vi "Execute Subscription Policy.vi"(9 "Publish Time":timestamp, 10 "New Topic Value":variant, 11 "Subscription Policy":T1) -> (0 "error out (Unsubscribe?)":errorcluster, 3 "Subscription Policy Out":T1)   [LabVIEW 2017, in "IMediator.lvlib" / "ISubscriptionPolicy.lvclass"]
doc: "This method decides whether or not to send or otherwise handle the new data value. The policy is set and maintained by the subscriber. The Topic Actor knows no policy details, it just passes the new value in. If there is a failure inside this method, the Topic Actor must assume the listener is no longer valid (dead/unrecoverable) and should delete it from the Subscriber list.\n\n<License>\nCopyright © 2017 Composed Systems, LLC | All rights reserved\nwww.composed.io\n\nAuthor: Ethan Stern <ethan.stern@composed.io>\n\nThis software is provided \"AS IS\" WITHOUT WARRANTIES, either express or implied, AND IS FOR EDUCATIONAL PURPOSES ONLY.\n</License>"
uses:
  ISubscriptionPolicy.lvclass
  ISubscriptionPolicy Reference.ctl
  ISubscriptionPolicy.lvclass/ISubscriptionPolicy.ctl
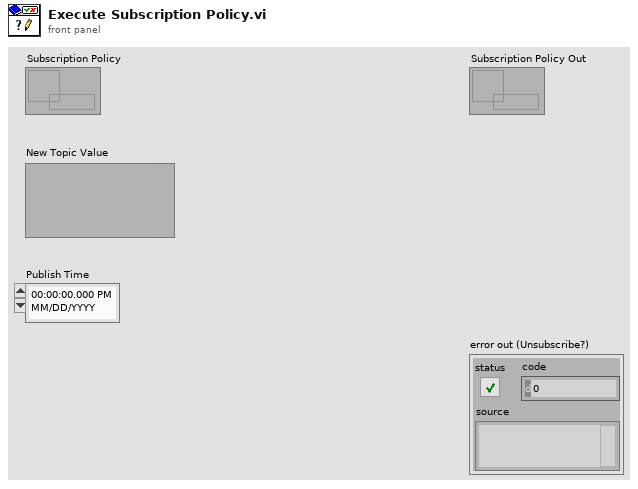
[diagram p1: front panel]
types:
  T1 = typedef "IMediator.lvlib/ISubscriptionPolicy.lvclass/ISubscriptionPolicy Reference.ctl" = refnum<data-value>
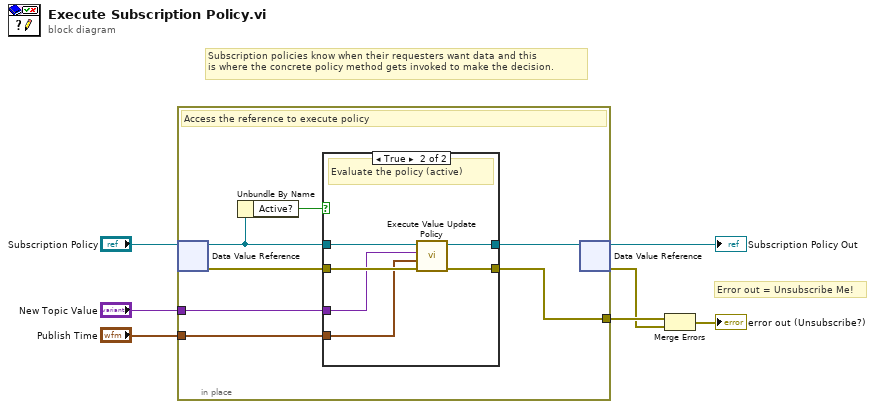
[diagram p0: block diagram]
diagram:
  # "Error out = Unsubscribe Me!"
  # "Subscription policies know when their requesters want data and this\nis where the concrete policy method gets invoked to make the decision."
  n1 = in-place {
    in-place-border: "New Topic Value" -> [w12]
    in-place-border: "Publish Time" -> [w11]
    in-place-border: [w10] -> w4
    # "Access the reference to execute policy"
    n2 = in-place-dvr #1("Subscription Policy") -> (w9:refnum<class "ISubscriptionPolicy.lvclass">, w13:errorcluster)
    n3 = Unbundle By Name(w9) -> ("Active?"=w8:bool)
    n4 = case shown="True" w8 {
      tunnel: w9 -> [w16 w22]
      tunnel: [w16 w21] -> w14
      tunnel: w13 -> [w15 w20]
      tunnel: w12 -> [_ w19]
      tunnel: w11 -> [_ w18]
      tunnel: [w15 w17] -> w10
      frame False {
        # "Skip evaluation (not active)"
      }
      frame True {
        # "Evaluate the policy (active)"
        n5 = call-dynamic "Execute Value Update Policy.vi"("error in (no error)"=w20, "Publish Time"=w18, "New Topic Value"=w19, "ISubscriptionPolicy In"=w22) -> ("error out"=w17:errorcluster, "ISubscriptionPolicy Out"=w21:refnum<class "ISubscriptionPolicy.lvclass">)  [unwired: 6 in]
      }
    }
    n6 = in-place-dvr #1(w14) -> (→"Subscription Policy Out":T1, w3:errorcluster)
  }
  n7 = Merge Errors(w4, w3) -> (→"error out (Unsubscribe?)":errorcluster)
